vi "go to load fuel.vi"(0 "system status in":T2={"system state"=enum."Empty & Closed", "fuel level"=0.0, "LOX level"=0.0, "system warnings"={"oxidizer overpress"=FALSE, "oxidizer leak"=FALSE, "fuel overpress"=FALSE, "fuel leak"=FALSE}, "valves"={"fuel load"=FALSE, "fuel return"=FALSE, "fuel comb"=FALSE, "fuel dump"=FALSE, "LOX load"=FALSE, "LOX return"=FALSE, "LOX comb"=FALSE, "LOX dump"=FALSE}, "ignition"=FALSE}, 11 "rocket controls":T1) -> (4 "system status out":T2={"system state"=enum."Empty & Closed", "fuel level"=0.0, "LOX level"=0.0, "system warnings"={"oxidizer overpress"=FALSE, "oxidizer leak"=FALSE, "fuel overpress"=FALSE, "fuel leak"=FALSE}, "valves"={"fuel load"=FALSE, "fuel return"=FALSE, "fuel comb"=FALSE, "fuel dump"=FALSE, "LOX load"=FALSE, "LOX return"=FALSE, "LOX comb"=FALSE, "LOX dump"=FALSE}, "ignition"=FALSE})   [LabVIEW 2017]
doc: "This subVI handles the logic going to the load fuel state for the rocket engine simulation.\nIt sets the state enum to the load fuel state when the load fuel button is pushed and thye fuel tank level is less than 100. \n\nPaul K Dixon\nP350\nCSUSB"
uses:
  typedefs/sysyem status.ctl
  typedefs/system state.ctl
  typedefs/rocket system warnings.ctl
  typedefs/user controls.ctl
panel:
  # "Standard\nProcedures"
  # "Alternate\nProcedures"
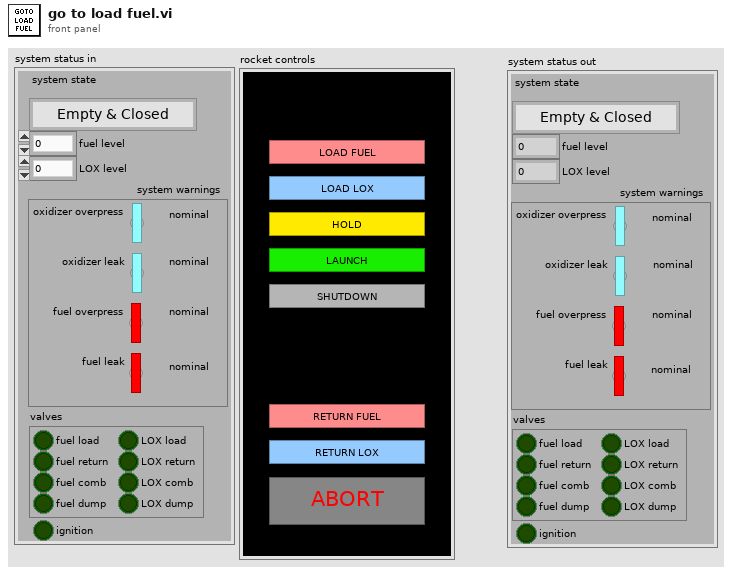
[diagram p1: front panel]
types:
  T1 = typedef "user controls.ctl" = cluster{"load fuel":bool, "load lox":bool, "hold":bool, "launch":bool, "shutdown":bool, "return fuel":bool, "return lox":bool, "abort":bool}
  T2 = typedef "sysyem status.ctl" = cluster{"system state":T3, "fuel level":dbl, "LOX level":dbl, "system warnings":T4, "valves":cluster{"fuel load":bool, "fuel return":bool, "fuel comb":bool, "fuel dump":bool, "LOX load":bool, "LOX return":bool, "LOX comb":bool, "LOX dump":bool}, "ignition":bool}
  T3 = typedef "system state.ctl" = enum16{"Hold", "Empty & Closed", "Launch", "Return Fuel", "Return LOX", "Loading Lox", "Loading Fuel", "Shutdown", "Abort"}
  T4 = typedef "rocket system warnings.ctl" = cluster{"oxidizer overpress":bool, "oxidizer leak":bool, "fuel overpress":bool, "fuel leak":bool}
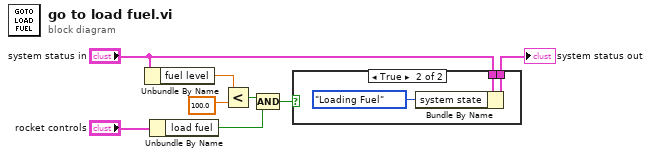
[diagram p0: block diagram]
diagram:
  n1 = Unbundle By Name("system status in") -> ("fuel level"=w2:dbl)
  n2 = Unbundle By Name("rocket controls") -> ("load fuel"=w7:bool)
  n3 = Less?(x=w2, y=100.0 ("x")) -> (x < y?=w6:bool)
  n4 = Compound Arithmetic op=AND(w6, w7) -> (w8:bool)
  n5 = case shown="True" w8 {
    tunnel: "system status in" -> [w9 w12]
    tunnel: [w9 w11] -> w4
    frame False {
    }
    frame True {
      n6 = Bundle By Name(cluster=w12, "system state"=system_state."Loading Fuel") -> (w11:T2)
    }
  }
  "system status out" <- w4
